vi "Get FP Conc.vi"(8 "error in":errorcluster, 11 "CPC in":refnum<class "CPC.lvclass">) -> (0 "error out":errorcluster, 2 "Conc":dbl, 3 "CPC out":refnum<class "CPC.lvclass">)   [LabVIEW 2014, in "CPC.lvclass"]
doc: "Read the concentration as displayed on the front panel. The concentration may have been derived from the photometric calibration, single-particle counting or live-time counting."
uses:
  CPC.lvclass
  Controls/3022A/Enum Cmd.ctl
  3022A/3022A.lvclass
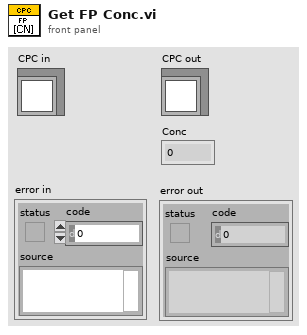
[diagram p1: front panel]
types:
  T1 = typedef "3022A.lvclass/Enum Cmd.ctl" = enum8{"CALIBRATE", "GET CAL DATA", "DUMP", "ESCAPE", "ID CAL LABEL", "INPUT CAL LABEL", "LIQUID LEVEL", "CONDENSER T", "SATURATOR T", "OPTICS T", "GET FLOW RATE", "READ ENV", "READ REF DETECTOR", "READ DETECTOR V", "READ 200 s BUFFER", "READ 20 s BUFFER", "READ 2 s BUFFER", "READ 1 s BUFFER", "READ PHOTOMETRIC CONC", "READ FP CONC", "READ MICROPROCESSOR PUMP CTL", "SENSOR", "SET VOLTAGE", "WRITE DISP MSG", "LASER OFF", "LASER ON", "PUMP OFF", "PUMP ON", "DRAIN", "FILL", "RESET CONC BUFFERS", "LOW FLOW MODE", "HIGH FLOW MODE"}
  T2 = cluster{"Cmd":T1, "x":i64, "y":i64, "Display":string}
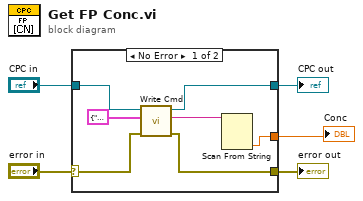
[diagram p0: block diagram]
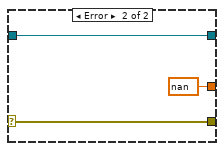
[diagram p2: hidden frame]
diagram:
  n1 = case shown="No Error" "error in" {
    selector: "error in" -> [w12 w15]
    tunnel: [w11 w15] -> w4
    tunnel: [w9 w14] -> w2
    tunnel: "CPC in" -> [w10 w14]
    tunnel: [w6 nan] -> w1
    frame No Error {
      n2 = call-dynamic "Write Cmd.vi"("error in"=w12, "CmdStruct"=T2 {"Cmd"=enum."READ FP CONC", "x"=0, "y"=0, "Display"=""}, "CPC in"=w10) -> ("error out"=w11:errorcluster, "Buffer"=w7:string, "CPC out"=w9:refnum<class "CPC.lvclass">)  [unwired: 6 in]
      n3 = Scan From String(input string=w7) -> (output 1=w6:dbl)  [unwired: 4 in, 3 out]
    }
    frame Error {
    }
  }
  "error out" <- w4
  "CPC out" <- w2
  "Conc" <- w1
